vi "PulseIn.vi"() -> ()   [LabVIEW 2015]
uses:
  <vilib>/rvi/eio/common/nirviEmuTemplateMethod_errors.vi
  <vilib>/eio/EIONode/EIONode.xnode
panel:
  out "US FL":i16
  out "US BK":i16
  out "US FR":i16
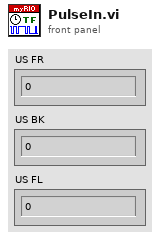
[diagram p1: front panel]
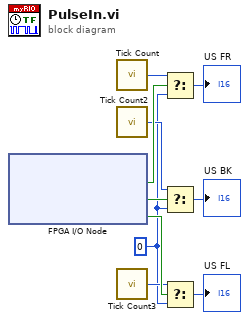
[diagram p0: block diagram]
diagram:
  w4 = i16 0
  n1 = xnode "FPGA I/O Node"() -> ("ConnectorA/DIO6"=w10:bool, "ConnectorA/DIO7"=w9:bool, "ConnectorA/DIO9"=w8:bool)  [unwired: 3 in, 3 out]
  n2 = call "Tick Count"() -> ("Tick Count(uSec)"=w7:u32)
  n3 = call "Tick Count2"() -> ("Tick Count(uSec)"=w6:u32)
  n4 = call "Tick Count3"() -> ("Tick Count(uSec)"=w5:u32)
  n5 = Select(t=w7, s=w10, f=w4) -> (s? t:f=→"US FR":u32)
  n6 = Select(t=w6, s=w9, f=w4) -> (s? t:f=→"US BK":u32)
  n7 = Select(t=w5, s=w8, f=w4) -> (s? t:f=→"US FL":u32)
